vi "TrapProfile_TotalTime.vi"(11 "TRAPEZOID_PROFILE":T1 {"Goal"."Velocity" format="%16_6e"; "Goal"."Position" format="%16_6e"; "Initial"."Velocity" format="%16_6e"; "Initial"."Position" format="%16_6e"; "Constraints"."MaxAcceleration" format="%16_6e"; "Constraints"."MaxVelocity" format="%16_6e"; "EndDecel" format="%16_6e"; "EndFullSpeed" format="%16_6e"; "EndAccel" format="%16_6e"}) -> (3 "TotalTime":dbl)   [LabVIEW 2019, in "Trajectory_Library.lvlib"]
doc: "Returns the total time the profile takes to reach the goal.\n \nInputs:\n - Trapezoid_Profile -- The Trapezoid_Profile data cluster\n\nOutputs:\n - TotalTime -- Total time to reach goal (seconds)"
uses:
  Trajectory_Library.lvlib
  TypeDef/TRAPEZOID_PROFILE.ctl
  TypeDef/TRAPEZOID_PROFILE_CONSTRAINT.ctl
  TypeDef/TRAPEZOID_PROFILE_STATE.ctl
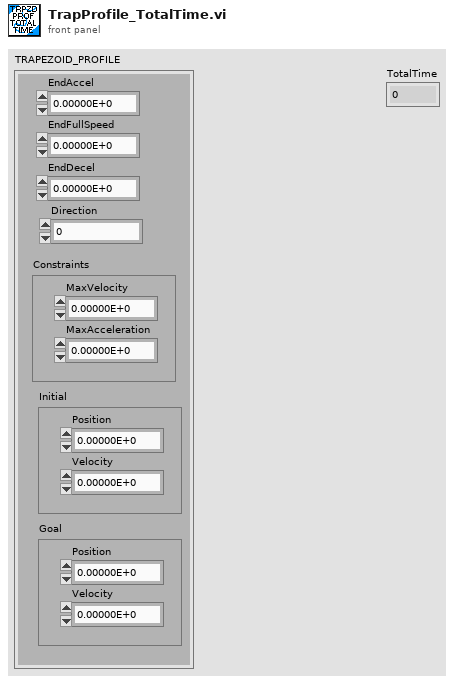
[diagram p1: front panel]
types:
  T1 = typedef "Trajectory_Library.lvlib/TRAPEZOID_PROFILE.ctl" = cluster{"EndAccel":dbl, "EndFullSpeed":dbl, "EndDecel":dbl, "Direction":i32, "Constraints":T2, "Initial":T3, "Goal":T3}
  T2 = typedef "Trajectory_Library.lvlib/TRAPEZOID_PROFILE_CONSTRAINT.ctl" = cluster{"MaxVelocity":dbl, "MaxAcceleration":dbl}
  T3 = typedef "Trajectory_Library.lvlib/TRAPEZOID_PROFILE_STATE.ctl" = cluster{"Position":dbl, "Velocity":dbl}
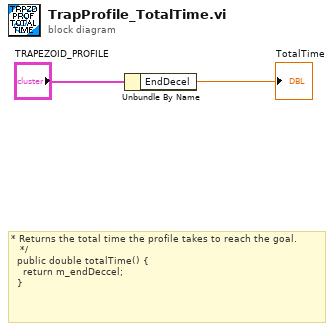
[diagram p0: block diagram]
diagram:
  # "* Returns the total time the profile takes to reach the goal.\n   */\n  public double totalTime() {\n    return m_endDeccel;\n  }"
  n1 = Unbundle By Name("TRAPEZOID_PROFILE") -> ("EndDecel"=→"TotalTime":dbl)
